vi "SP Calibration Debugging Tool.vi"(0 "Case 1":bool, 1 "Parameters to Measure":T3[](array[typedef]) {"Channel" min=1 max=99 step=1; "Parameter"."Stimulus Port" min=1 step=1; "Parameter"."Response Port" min=1 step=1}, 2 "Previous Info":string, 5 "Stimulus Changing? (f)":bool, 7 "!= Not Calibrated":bool, 9 "Case 2":bool, 11 "Action":T1(ring), 12 "Current Cal state":T2, 13 "Action 2":T1(ring)) -> ()   [LabVIEW 2011]
uses:
  TypeDefs/SP Parameter to Measure.ctl
  TypeDefs/SP Parameter.ctl
  TypeDefs/SP Calibration State.ctl
  TypeDefs/SP Measurement Format.ctl
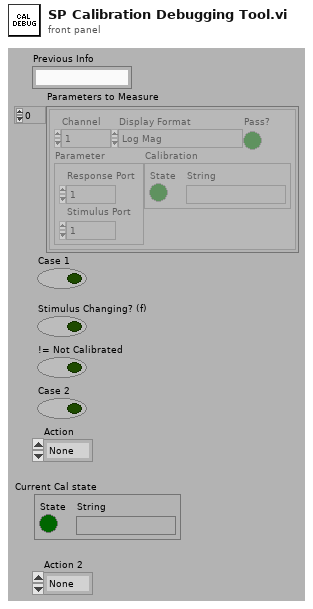
[diagram p1: front panel]
types:
  T1 = enum16{"None", "Calibrate", "Restore", "Ignore", "Abort"}
  T2 = typedef "SP Calibration State.ctl" = cluster{"State":bool, "String":string}
  T3 = typedef "SP Parameter to Measure.ctl" = cluster{"Channel":i8, "Parameter":T4, "Calibration":T2, "Display Format":T5, "Pass?":bool}
  T4 = typedef "SP Parameter.ctl" = cluster{"Stimulus Port":i8, "Response Port":i8}
  T5 = typedef "SP Measurement Format.ctl" = enum32{"Log Mag", "Phase", "Delay", "Smith (R+jX)", "Polar (Re/Im)", "Linear Mag", "SWR", "Real", "Imaginary", "Smith (Lin/Phase)", "Smith (Log/Phase)", "Smith (Real/Imag)", "Smith (G+jB)", "Polar (Lin/Phase)", "Polar (Log/Phase)", "Expanded Phase", "Positive Phase", "Inverted Smith", "Unwrapped Phase", "Power Out", "Power In", "Linear Mag/Phase", "Log Mag/Phase", "Real/Imaginary"}
  T6 = enum32{"invalid app kind", "Development System", "Run Time System", "Student Edition", "Embedded LabVIEW", "Evaluation", "Custom"}
  T7 = enum16{"open", "replace", "create", "open or create", "replace or create", "replace or create with confirmation"}
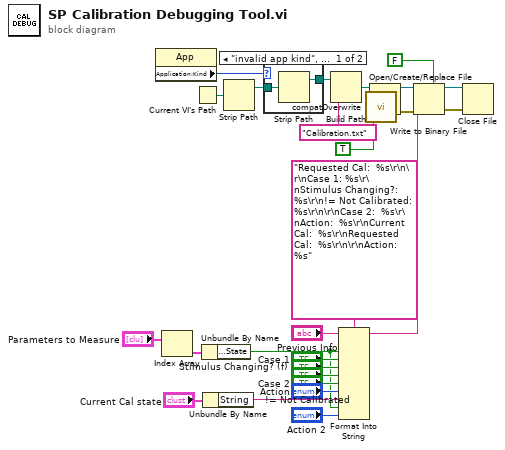
[diagram p0: block diagram]
diagram:
  n1 = property class="App"() -> ("Application:Kind"=w9:T6)  [unwired: 2 in, 2 out]
  n2 = Index Array(array="Parameters to Measure") -> (element=w6:T3)  [unwired: 1 in]
  n3 = Current VI's Path() -> (path=w13:path)
  n4 = Unbundle By Name(w6) -> ("Calibration.State"=w5:bool)
  n5 = Unbundle By Name("Current Cal state") -> ("String"=w1:string)
  n6 = Strip Path(path=w13) -> (stripped path=w11:path)  [unwired: 1 out]
  n7 = case shown="\"invalid app kind\", Default" w9 {
    tunnel: w11 -> [w29 w30]
    tunnel: [w28 w30] -> w10
    frame "invalid app kind", Default {
      n8 = Strip Path(path=w29) -> (stripped path=w28:path)  [unwired: 1 out]
    }
    frame "Development System" {
    }
  }
  n9 = Build Path(base path=w10, name or relative path="Calibration.txt") -> (appended path=w8:path)
  n10 = Format Into String(format string="Requested Cal:  %s\r\n\r\nCase 1: %s\r\nStimulus Changing?:  %s\r\n!= Not Calibrated:  %s\r\n\r\nCase 2:  %s\r\nAction:  %s\r\nCurrent Cal:  %s\r\nRequested Cal:  %s\r\n\r\nAction:  %s", initial string="Previous Info", w5, "Case 1", "Stimulus Changing? (f)", "!= Not Calibrated", "Case 2", "Action", w1, w5, "Action 2") -> (resulting string=w26:string)  [unwired: 1 in, 1 out]
  n11 = call <vilib>:"compatOverwrite.vi"("overwrite (F)"=TRUE) -> ("overwrite?"=w3:T7)
  n12 = Open/Create/Replace File(file path (use dialog)=w8, operation (0:open)=w3) -> (refnum out=w14:refnum<file>, error out=w17:errorcluster)  [unwired: 1 in, 4 out]
  n13 = Write to Binary File(file (use dialog)=w14, data=w26, error in=w17, 5:FALSE ("prepend array or string size? (T)")) -> (refnum out=w15:refnum<file>, error out=w16:errorcluster)  [unwired: 3 out]
  n14 = Close File(refnum=w15, error in=w16) -> ()  [unwired: 2 out]
